vi "Icon_Calculate Size Rule.vi"(8 "Error":errorcluster, 9 "Text Size":i32, 11 "Rows":u32) -> (0 "Error Out":errorcluster, 3 "Rule Out":T1)   [LabVIEW 2009]
uses:
  Controls/Enum/ENUM_Icon Sizing.ctl
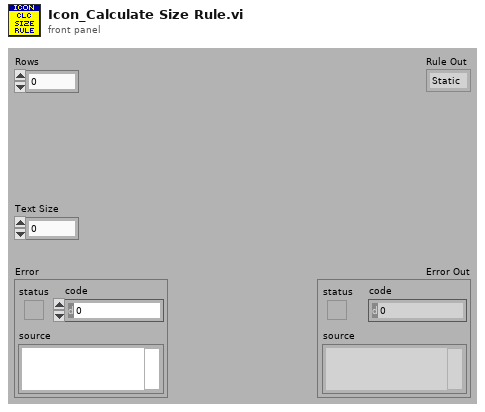
[diagram p1: front panel]
types:
  T1 = typedef "ENUM_Icon Sizing.ctl" = enum16{"Static", "Auto"}
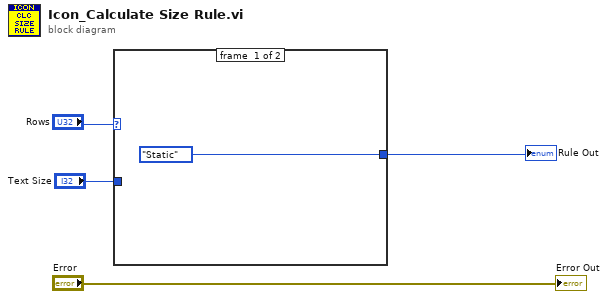
[diagram p0: block diagram]
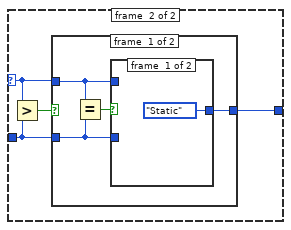
[diagram p2: hidden frame]
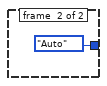
[diagram p3: hidden frame]
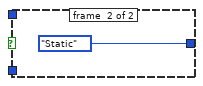
[diagram p4: hidden frame]
diagram:
  n1 = case shown="..4" "Rows" {
    selector: "Rows" -> [_ w6]
    tunnel: [ENUM_Icon_Sizing."Static" ("Rule") w9] -> w4
    tunnel: "Text Size" -> [_ w7]
    frame #0 {
    }
    frame #1 {
      n2 = Greater?(x=w6, y=w7) -> (0:w8:bool)
      n3 = case shown="True" w8 {
        tunnel: w6 -> [w10 _]
        tunnel: w7 -> [w11 _]
        tunnel: [w12 ENUM_Icon_Sizing."Static" ("Rule")] -> w9
        frame #0 {
          n4 = Equal?(x=w10, y=w11) -> (x = y?=w13:bool)
          n5 = case shown="True" w13 {
            tunnel: [ENUM_Icon_Sizing."Static" ("Rule") ENUM_Icon_Sizing."Auto" ("Rule")] -> w12
            tunnel: w11 -> [_ _]
            tunnel: w10 -> [_ _]
            frame #0 {
            }
            frame #1 {
            }
          }
        }
        frame #1 {
        }
      }
    }
  }
  "Rule Out" <- w4
  "Error Out" <- "Error"
